vi "ORS_Fit_Recalibration_Fringes.vi"(0 "polynomial order":i32=2, 1 "n Recalibration Fringes":dbl[][](array[numeric]), 5 "polynomial fit algorithm":T1(ring), 7 "moving average half width":i32=1, 9 "interpolation method":i32(ring)=2 items=["nearest", "linear", "spline", "cubic Hermite", "Lagrange"], 12 "Offset":i32, 14 "Length":i32) -> (6 "phase":dbl[](array[numeric]) format="%0.2f", 10 "inverted phase":dbl[](array[numeric]) format="%0.2f", 15 "rel.phase error":dbl[](array[numeric]) format="%0.2f")   [LabVIEW 2016]
uses:
  <vilib>/Analysis/baseanly.llb/Mean (DBL).vi
  <vilib>/Analysis/3filter.llb/IIR Filter (DBL).vi
  <vilib>/Analysis/NI_AALPro.lvlib
  <vilib>/ptbypt/NI_PtbyPt.lvlib
  <vilib>/gmath/NI_Gmath.lvlib
  <vilib>/Analysis/NI_AALBase.lvlib
panel:
  out "Mean fringes":dbl[][](graph)
  out "Unwrapped Hilbert phase":dbl[][](graph)
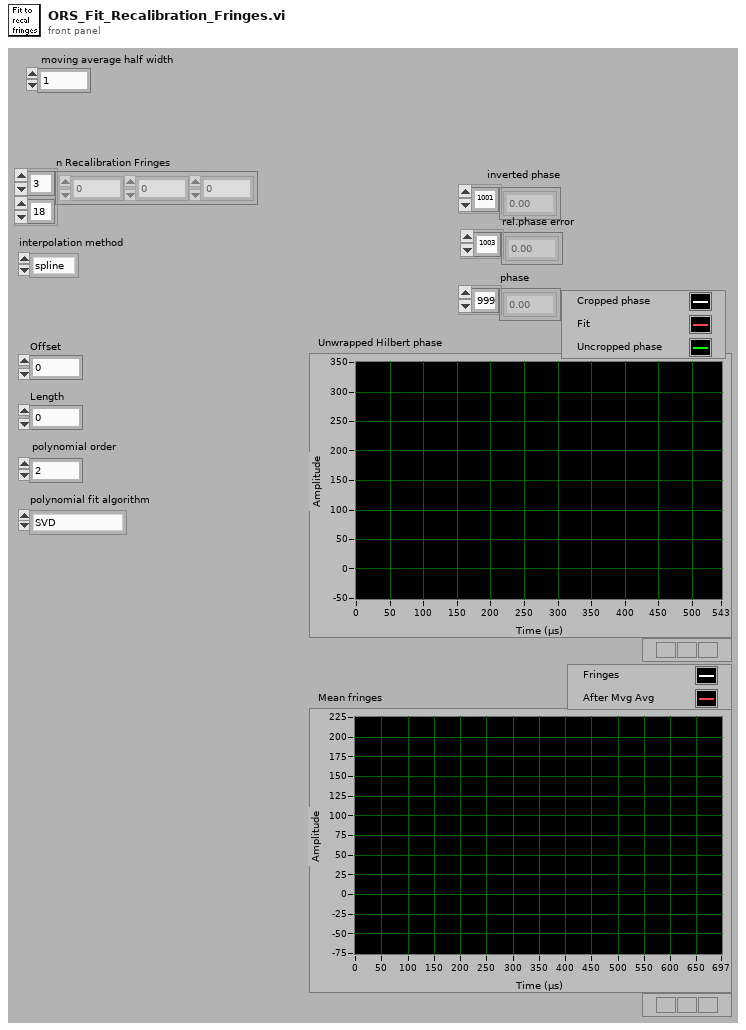
[diagram p1: front panel]
types:
  T1 = enum32{"SVD", "Givens", "Givens2", "Householder", "LU Decomposition", "Cholesky"}
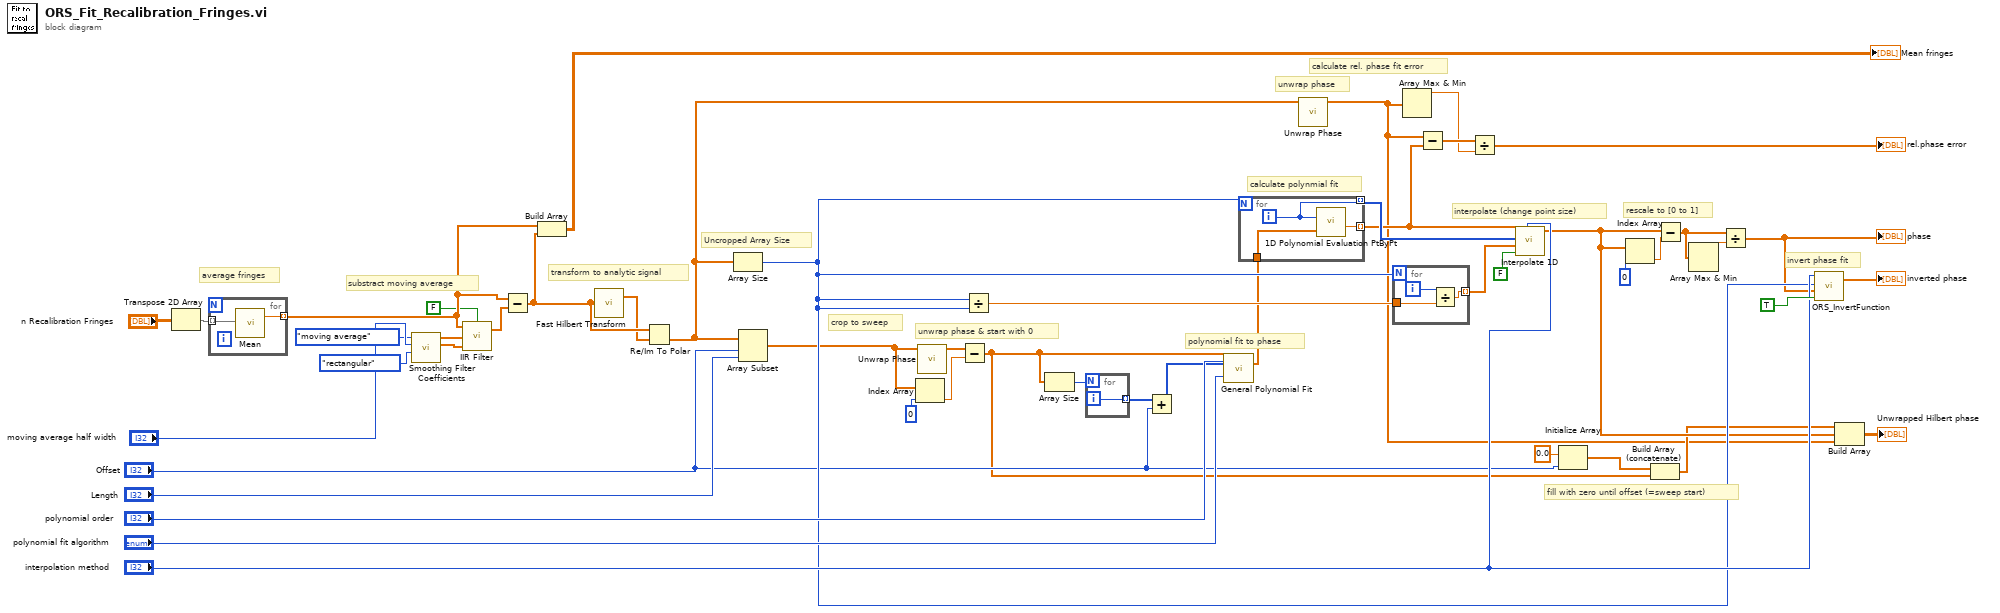
[diagram p0: block diagram]
diagram:
  # "transform to analytic signal"
  # "unwrap phase"
  # "average fringes"
  # "fill with zero until offset (=sweep start)"
  # "unwrap phase & start with 0"
  # "Uncropped Array Size"
  # "calculate rel. phase fit error"
  # "rescale to [0 to 1]"
  # "interpolate (change point size)"
  # "calculate polynmial fit"
  # "polynomial fit to phase"
  # "substract moving average"
  # "invert phase fit"
  # "crop to sweep"
  n1 = Transpose 2D Array(2D array="n Recalibration Fringes") -> (transposed array=w30:dbl[][])
  n2 = for {
    tunnel: w30 -> [w52] mode=indexing
    tunnel: [w51] -> w14 mode=indexing
    n3 = call-poly <vilib>:"Mean.vi"("X"=w52) -> ("mean"=w51:dbl)  [unwired: 1 out]
  }
  n4 = call <vilib>:"Smoothing Filter Coefficients.vi"("shape"=enum16{"rectangular", "triangular"}."rectangular" ("filter shape"), "half-width"="moving average half width", "type"=enum16{"moving average", "exponential"}."moving average") -> ("forward coefficients"=w4:dbl[], "reverse coefficients"=w3:dbl[])  [unwired: 6 in, 1 out]
  n5 = call-poly <vilib>:"IIR Filter.vi"("init/cont (init:F)"=FALSE, "Forward Coefficients"=w4, "Reverse Coefficients"=w3, "X"=w14) -> ("Filtered X"=w2:dbl[])  [unwired: 1 out]
  n6 = Subtract(x=w14, y=w2) -> (x-y=w8:dbl[])
  n7 = Build Array(w14, w8) -> (→"Mean fringes":dbl[][])
  n8 = call <vilib>:"Fast Hilbert Transform.vi"("X"=w8) -> ("Hilbert{X}"=w1:dbl[])  [unwired: 1 out]
  n9 = Re/Im To Polar(2:w1, 3:w8) -> (0:w19:dbl[])  [unwired: 1 out]
  n10 = Array Size(array=w19) -> (size(s)=w33:i32)
  n11 = Array Subset(array=w19, index="Offset", length="Length") -> (w16:dbl[])
  n12 = Index Array(array=w16, index=0) -> (element=w20:dbl)
  n13 = call <vilib>:"Unwrap Phase.vi"("Phase"=w16) -> ("Unwrapped Phase"=w15:dbl[])  [unwired: 9 in, 1 out]
  n14 = Subtract(x=w15, y=w20) -> (x-y=w9:dbl[])
  n15 = Divide(x=w33, y=w33) -> (x/y=w32:dbl)
  n16 = Array Size(array=w9) -> (size(s)=w42:i32)
  n17 = for {
    N: w42 -> [_]
    tunnel: [w53] -> w41 mode=indexing
    i -> [w53]
  }
  n18 = Add(x=w41, y="Offset") -> (x+y=w40:i32[])
  n19 = call <vilib>:"General Polynomial Fit.vi"("Y"=w9, "polynomial order"="polynomial order", "X"=w40, "algorithm"="polynomial fit algorithm") -> ("Polynomial Coefficients"=w31:dbl[])  [unwired: 8 in, 3 out]
  n20 = for {
    N: w33 -> [_]
    tunnel: [w56] -> w28 mode=indexing
    tunnel: [w55] -> w43 mode=indexing
    tunnel: w31 -> [w54]
    i -> [w55]
    n21 = call <vilib>:"1D Polynomial Evaluation PtByPt.vi"("Coefficients: a"=w54, "x"=w55) -> ("y"=w56:dbl)
  }
  n22 = call <vilib>:"Unwrap Phase.vi"("Phase"=w19) -> ("Unwrapped Phase"=w17:dbl[])  [unwired: 9 in, 1 out]
  n23 = for {
    N: w33 -> [_]
    tunnel: [w57] -> w39 mode=indexing
    tunnel: w32 -> [w59]
    i -> [w58]
    n24 = Divide(x=w58, y=w59) -> (x/y=w57:dbl)
  }
  n25 = Array Max & Min(array=w17) -> (max value=w36:dbl)  [unwired: 3 out]
  n26 = Subtract(x=w17, y=w28) -> (x-y=w37:dbl[])
  n27 = Divide(x=w37, y=w36) -> (x/y=→"rel.phase error":dbl[])
  n28 = call <vilib>:"Interpolate 1D.vi"("method"="interpolation method", "X is monotonic"=FALSE, "xi"=w39, "X"=w43, "Y"=w28) -> ("yi"=w23:dbl[])  [unwired: 4 in, 2 out]
  n29 = Initialize Array(0.0 ("element"), "Offset") -> (w26:dbl[])
  n30 = Index Array(array=w23, index=0 ("Index")) -> (element=w48:dbl)
  n31 = Build Array (concatenate)(w26, w9) -> (w22:dbl[])
  n32 = Subtract(x=w23, y=w48) -> (x-y=w24:dbl[])
  n33 = Array Max & Min(array=w24) -> (max value=w46:dbl)  [unwired: 3 out]
  n34 = Divide(x=w24, y=w46) -> (x/y=w27:dbl[])
  "phase" <- w27
  n35 = call "ORS_InvertFunction.vi"("Rescale to input"=TRUE, "input"=w27, "number of points"=w33, "method"="interpolation method") -> ("inverted output"=→"inverted phase":dbl[])  [unwired: 1 in]
  n36 = Build Array(w22, w23, w17) -> (→"Unwrapped Hilbert phase":dbl[][])
